vi "global.vi"() -> ()   [LabVIEW 2018]
panel:
  out "Black":bool
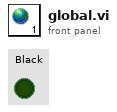
[diagram p1: front panel]
diagram:
